vi "Read Data Buffer.vi"(8 "error in (no error)":errorcluster, 11 "Calculation Worker in":refnum<class "Calculation Worker.lvclass">) -> (0 "error out":errorcluster, 2 "Data Buffer":T1, 3 "Calculation Worker out":refnum<class "Calculation Worker.lvclass">)   [LabVIEW 2020, in "Calculation Worker.lvlib" / "Calculation Worker.lvclass"]
uses:
  Calculation Worker.lvclass
  GPU FFT Calculator/GPU FFT Calculator/Data Source Buffer.ctl
  Calculation Worker.lvclass/Calculation Worker.ctl
  Data Source/Data Source/Data Source.lvclass
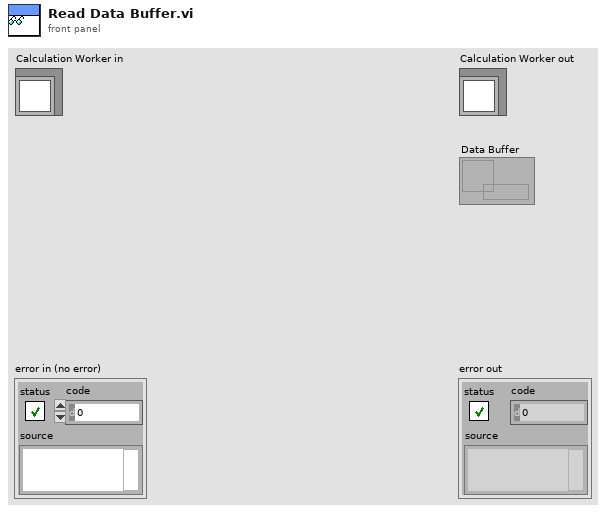
[diagram p1: front panel]
types:
  T1 = typedef "Data Source.lvlib/Data Source.lvclass/Data Source Buffer.ctl" = refnum<data-value>
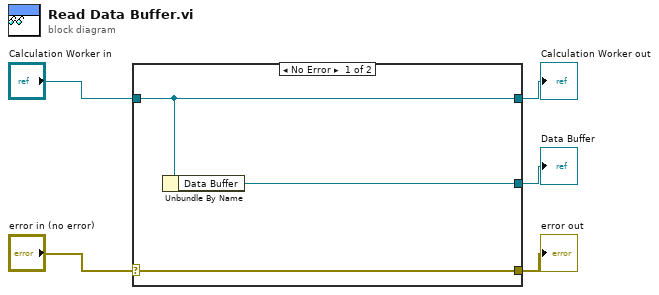
[diagram p0: block diagram]
diagram:
  n1 = case shown="No Error" "error in (no error)" {
    selector: "error in (no error)" -> [w8 w9]
    tunnel: [w8 w9] -> w4
    tunnel: [w7 w10] -> w2
    tunnel: "Calculation Worker in" -> [w7 w10]
    tunnel: [w6 _] -> w1
    frame No Error {
      n2 = Unbundle By Name(w7) -> ("Data Buffer"=w6:T1)
    }
    frame Error {
    }
  }
  "error out" <- w4
  "Calculation Worker out" <- w2
  "Data Buffer" <- w1
